vi "ZeroMQ_FOC_REQREP.vi"() -> ()   [LabVIEW 2018]
uses:
  <vilib>/addons/zeromq/socket_type.ctl
  <vilib>/addons/zeromq/socket_options.ctl
  <vilib>/addons/zeromq/zeromq.lvlib
  <vilib>/addons/zeromq/zmq_socket.lvclass
  <vilib>/addons/zeromq/zmq_context.lvclass
panel:
  out "error out 4":errorcluster
  in  "stop 4":bool
  out "command 2":string
  out "reply":string
  out "error out 2":errorcluster
  out "message":string
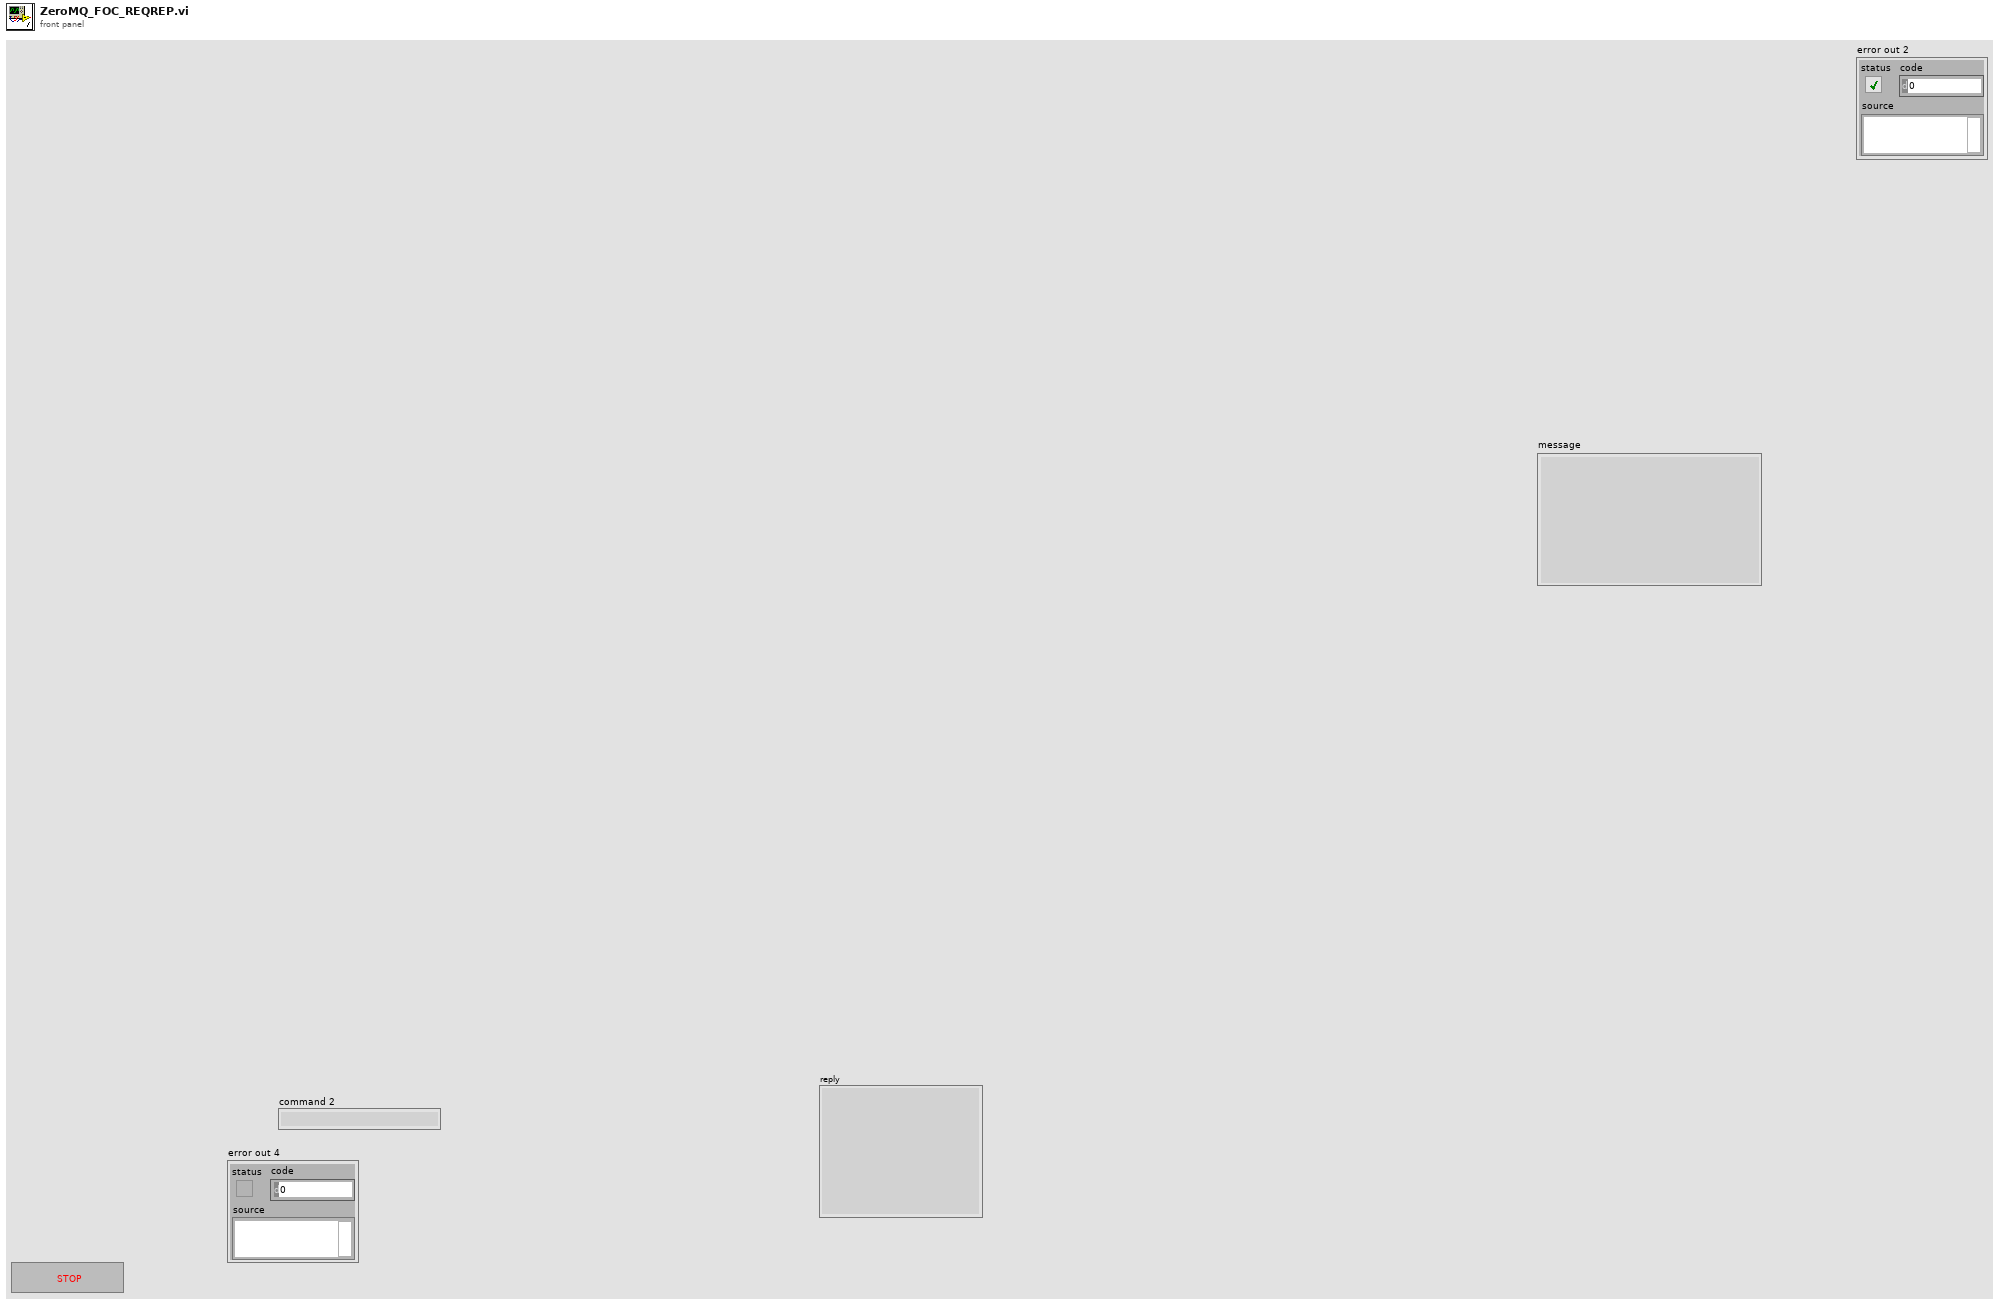
[diagram p1: front panel]
types:
  T1 = typedef "zeromq.lvlib/socket_options.ctl" = enum8{"NONE", "ZMQ_HWM", "<2>", "ZMQ_SWAP", "ZMQ_AFFINITY", "ZMQ_ROUTING_ID", "ZMQ_SUBSCRIBE", "ZMQ_UNSUBSCRIBE", "ZMQ_RATE", "ZMQ_RECOVERY_IVL", "ZMQ_MCAST_LOOP", "ZMQ_SNDBUF", "ZMQ_RCVBUF", "ZMQ_RCVMORE", "ZMQ_FD", "ZMQ_EVENTS", "ZMQ_TYPE", "ZMQ_LINGER", "ZMQ_RECONNECT_IVL", "ZMQ_BACKLOG", "ZMQ_RECOVERY_IVL_MSEC", "ZMQ_RECONNECT_IVL_MAX", "ZMQ_MAXMSGSIZE", "ZMQ_SNDHWM", "ZMQ_RCVHWM", "ZMQ_MULTICAST_HOPS", "<26>", "ZMQ_RCVTIMEO", "ZMQ_SNDTIMEO", "<29>", "<30>", "ZMQ_IPV4ONLY", "ZMQ_LAST_ENDPOINT", "ZMQ_ROUTER_MANDATORY", "ZMQ_TCP_KEEPALIVE", "ZMQ_TCP_KEEPALIVE_CNT", "ZMQ_TCP_KEEPALIVE_IDLE", "ZMQ_TCP_KEEPALIVE_INTVL", "ZMQ_TCP_ACCEPT_FILTER", "ZMQ_IMMEDIATE", "ZMQ_XPUB_VERBOSE", "ZMQ_ROUTER_RAW", "ZMQ_IPV6", "ZMQ_MECHANISM", "ZMQ_PLAIN_SERVER", "ZMQ_PLAIN_USERNAME", "ZMQ_PLAIN_PASSWORD", "ZMQ_CURVE_SERVER", "ZMQ_CURVE_PUBLICKEY", "ZMQ_CURVE_SECRETKEY", "ZMQ_CURVE_SERVERKEY", "ZMQ_PROBE_ROUTER", "ZMQ_REQ_CORRELATE", "ZMQ_REQ_RELAXED", "ZMQ_CONFLATE", "ZMQ_ZAP_DOMAIN", "ZMQ_ROUTER_HANDOVER", "ZMQ_TOS", "ZMQ_IPC_FILTER_PID", "ZMQ_IPC_FILTER_UID", "ZMQ_IPC_FILTER_GID", "ZMQ_CONNECT_ROUTING_ID", "ZMQ_GSSAPI_SERVER", "ZMQ_GSSAPI_PRINCIPAL", "ZMQ_GSSAPI_SERVICE_PRINCIPAL", "ZMQ_GSSAPI_PLAINTEXT", "ZMQ_HANDSHAKE_IVL", "<67>", "ZMQ_SOCKS_PROXY", "ZMQ_XPUB_NODROP", "ZMQ_BLOCKY", "ZMQ_XPUB_MANUAL", "ZMQ_XPUB_WELCOME_MSG", "ZMQ_STREAM_NOTIFY", "ZMQ_INVERT_MATCHING", "ZMQ_HEARTBEAT_IVL", "ZMQ_HEARTBEAT_TTL", "ZMQ_HEARTBEAT_TIMEOUT", "ZMQ_XPUB_VERBOSER", "ZMQ_CONNECT_TIMEOUT", "ZMQ_TCP_MAXRT", "ZMQ_THREAD_SAFE", "<82>", "<83>", "ZMQ_MULTICAST_MAXTPDU", "ZMQ_VMCI_BUFFER_SIZE", "ZMQ_VMCI_BUFFER_MIN_SIZE", "ZMQ_VMCI_BUFFER_MAX_SIZE", "ZMQ_VMCI_CONNECT_TIMEOUT", "ZMQ_USE_FD", "ZMQ_GSSAPI_PRINCIPAL_NAMETYPE", "ZMQ_GSSAPI_SERVICE_PRINCIPAL_NAMETYPE", "ZMQ_BINDTODEVICE", "ZMQ_ZAP_ENFORCE_DOMAIN", "ZMQ_LOOPBACK_FASTPATH", "ZMQ_METADATA", "ZMQ_MULTICAST_LOOP", "ZMQ_ROUTER_NOTIFY"}
  T2 = typedef "zeromq.lvlib/socket_type.ctl" = enum8{"ZMQ_PAIR", "ZMQ_PUB", "ZMQ_SUB", "ZMQ_REQ", "ZMQ_REP", "ZMQ_DEALER", "ZMQ_ROUTER", "ZMQ_PULL", "ZMQ_PUSH", "ZMQ_XPUB", "ZMQ_XSUB", "ZMQ_STREAM", "ZMQ_SERVER", "ZMQ_CLIENT", "ZMQ_RADIO", "ZMQ_DISH", "ZMQ_GATHER", "ZMQ_SCATTER", "ZMQ_DGRAM"}
  T3 = cluster{"ID":u32, "Address":string, "Service Name 1":string, "Service Name 2":string, "queue TX":refnum<queue>, "queue RX":refnum<queue>, "Port 1":u32, "Port 2":u32}
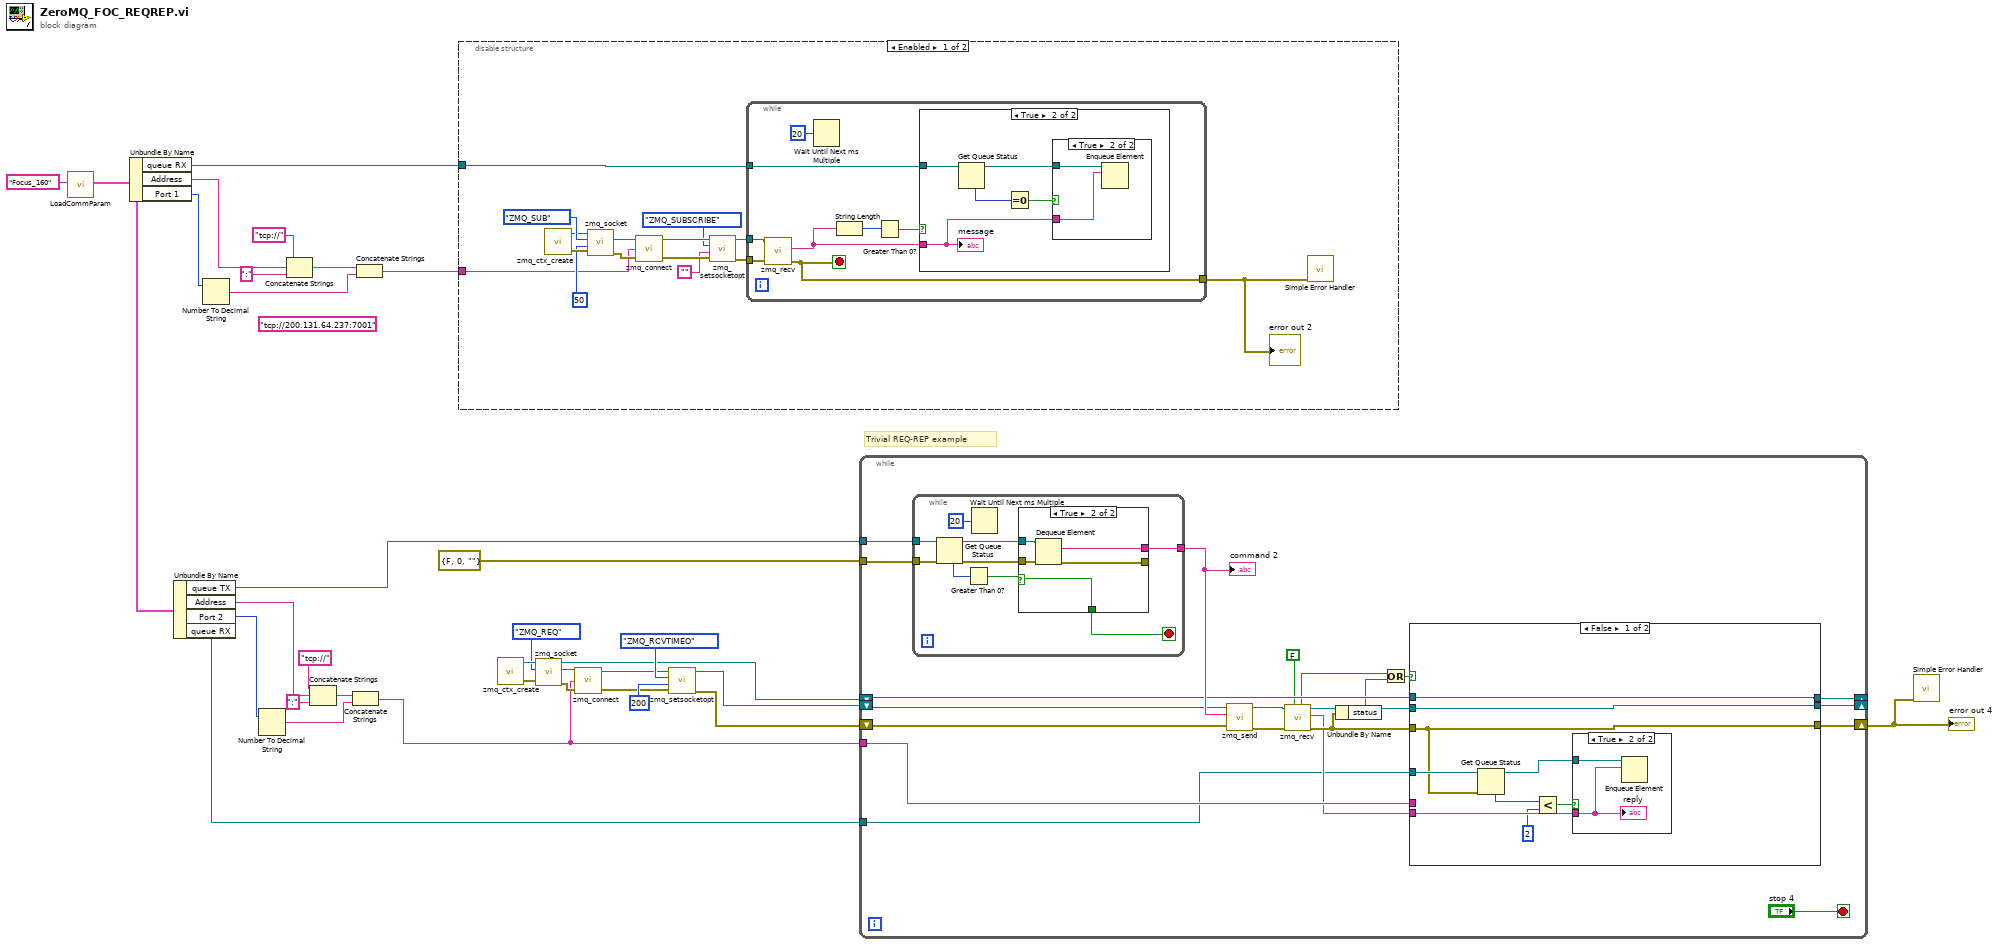
[diagram p0: block diagram]
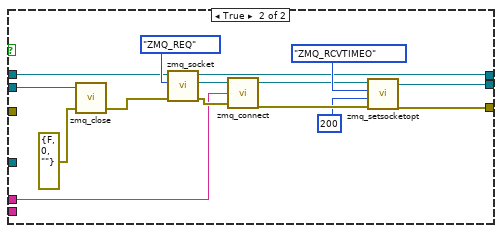
[diagram p3: hidden frame]
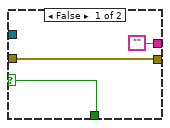
[diagram p4: hidden frame]
diagram:
  (unwired) "tcp://200.131.64.237:7001" ("endpoint")
  # "Trivial REQ-REP example"
  n1 = call "LoadCommParam.vi"("section name"="Focus_160") -> ("output cluster"=w1:T3)  [unwired: 10 in]
  n2 = Unbundle By Name(w1) -> ("queue RX"=w25:refnum<queue>, "Address"=w32:string, "Port 1"=w31:u32)
  n3 = Unbundle By Name(w1) -> ("queue TX"=w16:refnum<queue>, "Address"=w18:string, "Port 2"=w17:u32, "queue RX"=w2:refnum<queue>)
  n4 = Number To Decimal String(number=w31) -> (decimal integer string=w30:string)  [unwired: 1 in]
  n5 = Number To Decimal String(number=w17) -> (decimal integer string=w22:string)  [unwired: 1 in]
  n6 = Concatenate Strings("tcp://" ("string"), w32, ":" ("string")) -> (w29:string)
  n7 = Concatenate Strings("tcp://" ("string"), w18, ":" ("string")) -> (w21:string)
  n8 = Concatenate Strings(w21, w22) -> (w10:string)
  n9 = Concatenate Strings(w29, w30) -> (w26:string)
  n10 = disable-structure shown="Enabled" {
    disable-tunnel: w25 -> [w35 _]
    disable-tunnel: w26 -> [w34 _]
    frame Enabled {
      n11 = call <vilib>:"zmq_ctx_create.vi"() -> ("error out"=w47:errorcluster, "context out"=w37:refnum<class "zmq_context.lvclass">)  [unwired: 4 in]
      n12 = call <vilib>:"zmq_socket.vi"("error in"=w47, "linger (ms)"=50, "socket type"=socket_type."ZMQ_SUB", "context in"=w37) -> ("error out"=w46:errorcluster, "socket out"=w38:refnum<class "zmq_socket.lvclass">)  [unwired: 1 in, 1 out]
      n13 = call <vilib>:"zmq_connect.vi"("error in"=w46, "endpoint"=w34, "socket in"=w38) -> ("error out"=w44:errorcluster, "socket out"=w45:refnum<class "zmq_socket.lvclass">)  [unwired: 1 in]
      n14 = call <vilib>:"zmq_setsocketopt.vi"("error in"=w44, "value"="", "option"=socket_options."ZMQ_SUBSCRIBE", "socket in"=w45) -> ("error out"=w43:errorcluster, "socket out"=w42:refnum<class "zmq_socket.lvclass">)  [unwired: 2 in]
      n15 = while {
        tunnel: w42 -> [w54]
        tunnel: w43 -> [w56]
        tunnel: [w55] -> w39
        tunnel: w35 -> [w51]
        stop <- w55 stop-if-true
        n16 = call <vilib>:"zmq_recv.vi"("error in"=w56, "socket in"=w54) -> ("error out"=w55:errorcluster, "data"=w50:string)  [unwired: 3 in, 3 out]
        n17 = Wait Until Next ms Multiple(millisecond multiple=u32 20) -> ()  [unwired: 1 out]
        n18 = String Length(string=w50) -> (length=w53:i32)
        n19 = Greater Than 0?(x=w53) -> (x > 0?=w52:bool)
        n20 = case shown="True" w52 {
          tunnel: w51 -> [_ w60]
          tunnel: w50 -> [_ w57]
          frame False {
          }
          frame True {
            n21 = Get Queue Status(queue=w60) -> (queue out=w58:refnum<queue>, # elements in queue=w61:i32)  [unwired: 2 in, 6 out]
            n22 = Equal To 0?(x=w61) -> (x = 0?=w59:bool)
            n23 = case shown="True" w59 {
              tunnel: w58 -> [_ w63]
              tunnel: w57 -> [_ w62]
              frame False {
              }
              frame True {
                n24 = Enqueue Element(queue=w63, element=w62) -> ()  [unwired: 2 in, 3 out]
              }
            }
            "message" <- w57
          }
        }
      }
      "error out 2" <- w39
      n25 = call <vilib>:"Simple Error Handler.vi"("error in (no error)"=w39) -> ()  [unwired: 4 in, 5 out]
    }
    frame Disabled {
    }
  }
  n26 = call <vilib>:"zmq_ctx_create.vi"() -> ("error out"=w15:errorcluster, "context out"=w12:refnum<class "zmq_context.lvclass">)  [unwired: 4 in]
  n27 = call <vilib>:"zmq_socket.vi"("error in"=w15, "socket type"=socket_type."ZMQ_REQ", "context in"=w12) -> ("error out"=w13:errorcluster, "socket out"=w14:refnum<class "zmq_socket.lvclass">, "context out"=w5:refnum<class "zmq_context.lvclass">)  [unwired: 2 in]
  n28 = call <vilib>:"zmq_connect.vi"("error in"=w13, "endpoint"=w10, "socket in"=w14) -> ("error out"=w6:errorcluster, "socket out"=w7:refnum<class "zmq_socket.lvclass">)  [unwired: 1 in]
  n29 = call <vilib>:"zmq_setsocketopt.vi"("error in"=w6, "value"=200 ("max queue size (-1, unlimited)"), "option"=socket_options."ZMQ_RCVTIMEO", "socket in"=w7) -> ("error out"=w3:errorcluster, "socket out"=w4:refnum<class "zmq_socket.lvclass">)  [unwired: 2 in]
  n30 = while {
    tunnel: w16 -> [w84]
    tunnel: errorcluster {"status"=FALSE, "code"=0, "source"=""} ("error out") -> [w80]
    tunnel: w10 -> [w69]
    shift-right: [w68] -> _
    shift-left: w5 -> [w79]
    shift-right: [w67] -> _
    shift-left: w4 -> [w78]
    shift-right: [w81] -> w24
    shift-left: w3 -> [w66]
    tunnel: w2 -> [w64]
    stop <- "stop 4" stop-if-true
    n31 = while {
      tunnel: w84 -> [w118]
      tunnel: w80 -> [w117]
      tunnel: [w113] -> w83
      stop <- w112 stop-if-true
      n32 = Get Queue Status(queue=w118, error in (no error)=w117) -> (queue out=w114:refnum<queue>, error out=w115:errorcluster, # elements in queue=w119:i32)  [unwired: 1 in, 5 out]
      n33 = Greater Than 0?(x=w119) -> (x > 0?=w116:bool)
      n34 = Wait Until Next ms Multiple(millisecond multiple=u32 20) -> ()  [unwired: 1 out]
      n35 = case shown="True" w116 {
        selector: w116 -> [w120 w123]
        tunnel: w115 -> [w122 w127]
        tunnel: w114 -> [_ w126]
        tunnel: [w122 w125] -> _
        tunnel: ["" w124] -> w113
        tunnel: [w120 w123] -> w112
        frame False {
        }
        frame True {
          n36 = Dequeue Element(queue=w126, error in (no error)=w127) -> (element=w124:string, error out=w125:errorcluster)  [unwired: 1 in, 2 out]
        }
      }
    }
    "command 2" <- w83
    n37 = call <vilib>:"zmq_send.vi"("error in"=w66, "data"=w83, "socket in"=w78) -> ("error out"=w76:errorcluster, "socket out"=w77:refnum<class "zmq_socket.lvclass">)  [unwired: 4 in]
    n38 = call <vilib>:"zmq_recv.vi"("no block? (F)"=FALSE, "error in"=w76, "socket in"=w77) -> ("error out"=w71:errorcluster, "data"=w65:string, "socket out"=w70:refnum<class "zmq_socket.lvclass">, "timeout?"=w72:bool)  [unwired: 2 in, 1 out]
    n39 = Unbundle By Name(w71) -> ("status"=w73:bool)
    n40 = Or(x=w72, y=w73) -> (x .or. y?=w74:bool)
    n41 = case shown="False" w74 {
      tunnel: [w88 w98] -> w81
      tunnel: w79 -> [w92 w100]
      tunnel: w71 -> [w88 _]
      tunnel: w70 -> [w93 w101]
      tunnel: w69 -> [_ w99]
      tunnel: [w93 w97] -> w67
      tunnel: [w92 w96] -> w68
      tunnel: w65 -> [w90 _]
      tunnel: w64 -> [w89 _]
      frame False {
        n42 = Get Queue Status(queue=w89, error in (no error)=w88) -> (queue out=w91:refnum<queue>, # elements in queue=w86:i32)  [unwired: 1 in, 6 out]
        n43 = Less?(x=w86, y=2) -> (x < y?=w87:bool)
        n44 = case shown="True" w87 {
          tunnel: w91 -> [_ w95]
          tunnel: w90 -> [_ w94]
          frame False {
          }
          frame True {
            n45 = Enqueue Element(queue=w95, element=w94) -> ()  [unwired: 2 in, 3 out]
            "reply" <- w94
          }
        }
      }
      frame True {
        n46 = call <vilib>:"zmq_close.vi"("error in"=errorcluster {"status"=FALSE, "code"=0, "source"=""}, "socket"=w101) -> ("error out"=w103:errorcluster)  [unwired: 3 in]
        n47 = call <vilib>:"zmq_socket.vi"("error in"=w103, "socket type"=socket_type."ZMQ_REQ", "context in"=w100) -> ("error out"=w109:errorcluster, "socket out"=w110:refnum<class "zmq_socket.lvclass">, "context out"=w96:refnum<class "zmq_context.lvclass">)  [unwired: 2 in]
        n48 = call <vilib>:"zmq_connect.vi"("error in"=w109, "endpoint"=w99, "socket in"=w110) -> ("error out"=w105:errorcluster, "socket out"=w106:refnum<class "zmq_socket.lvclass">)  [unwired: 1 in]
        n49 = call <vilib>:"zmq_setsocketopt.vi"("error in"=w105, "value"=200 ("max queue size (-1, unlimited)"), "option"=socket_options."ZMQ_RCVTIMEO", "socket in"=w106) -> ("error out"=w98:errorcluster, "socket out"=w97:refnum<class "zmq_socket.lvclass">)  [unwired: 2 in]
      }
    }
  }
  "error out 4" <- w24
  n50 = call <vilib>:"Simple Error Handler.vi"("error in (no error)"=w24) -> ()  [unwired: 4 in, 5 out]
